vi "FTT Format data.vi"(8 "error in (no error)":errorcluster, 10 "FTT_TV":string, 11 "W/R":bool) -> (0 "error out":errorcluster, 2 "FTT_TV Out":string, 3 "Display":T1)   [LabVIEW 2014]
uses:
  Type'def/Main FTT.ctl
panel:
  # "Plan/Targe(%)"
  # "Taget/Actual"
  # "FTT/FTT(%)"
  # "Repaired/Reject"
  # "/"
  # "/"
  # "/"
  # "/"
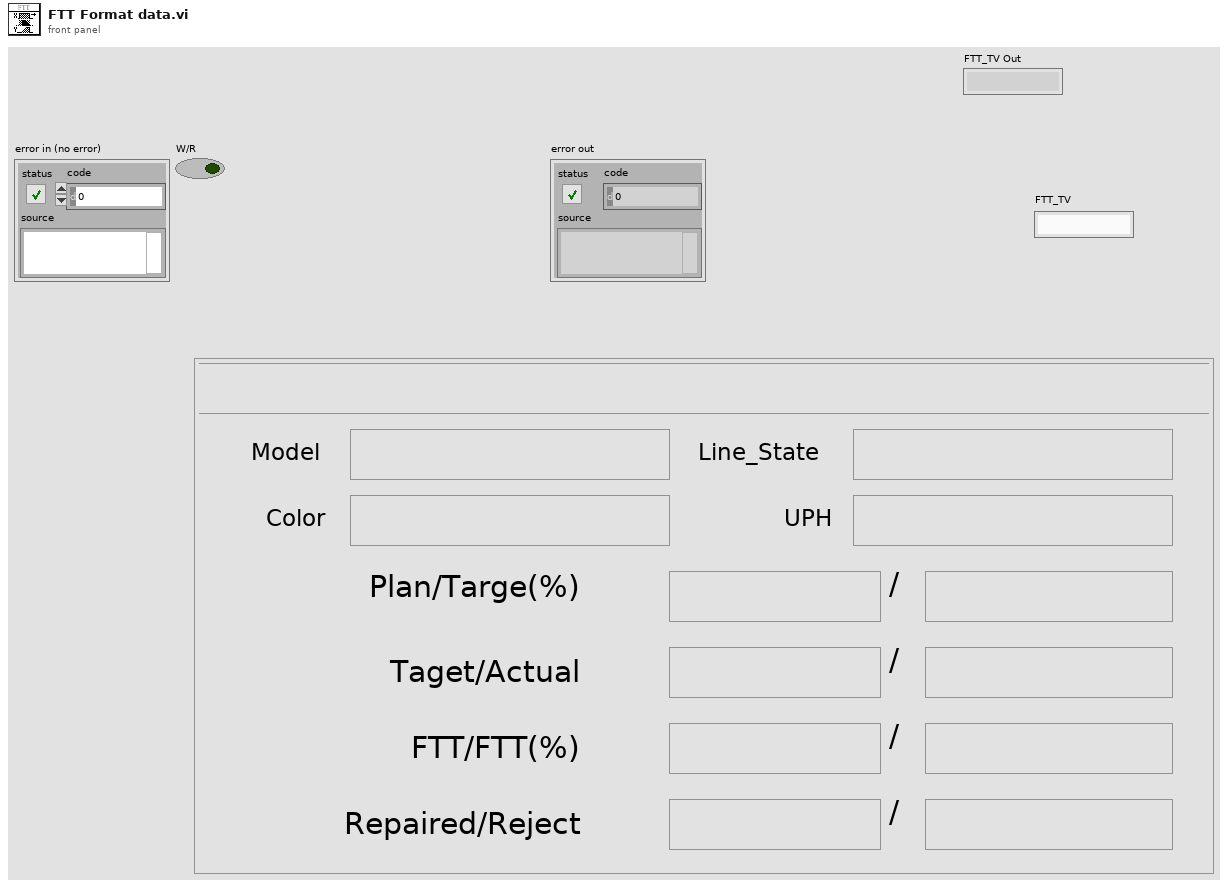
[diagram p1: front panel]
types:
  T1 = typedef "Main FTT.ctl" = cluster{"Line_Name":string, "Model":string, "Line_State":string, "Color":string, "UPH":string, "Plan":string, "Target Rate":string, "Target":string, "Actual":string, "FTT":string, "FTT Rate":string, "Repaired":string, "Reject":string}
  T2 = typedef "FTT Display Type.ctl" = cluster{"Line.No":string, "Model":string, "Color":string, "UPH":dbl, "Plan":dbl, "Target Rate":dbl, "Target ":dbl, "Actual":dbl, "FTT":dbl, "FTT Rate":dbl, "Repaired":dbl, "Reject":dbl, "Ouline":dbl, "Line State":string}
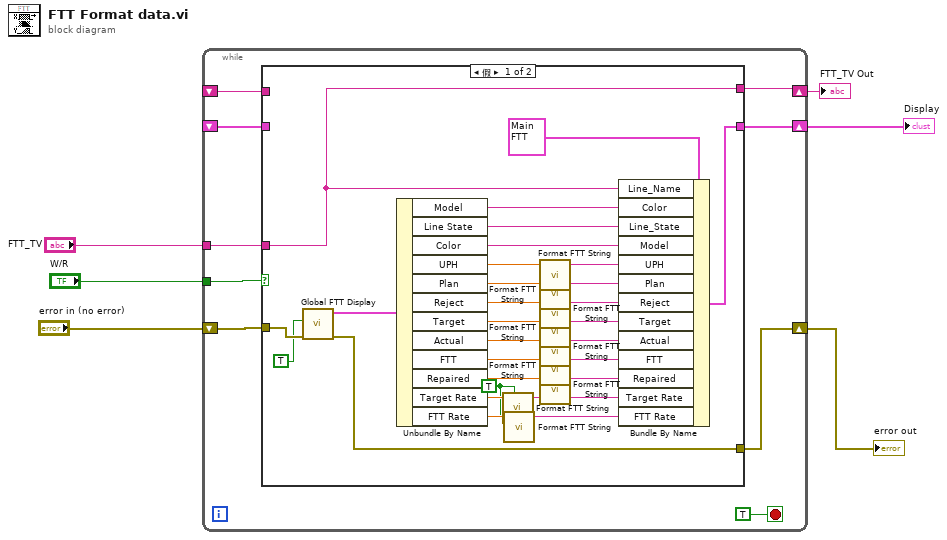
[diagram p0: block diagram]
diagram:
  n1 = while {
    shift-right: [w14] -> w5
    shift-left: "error in (no error)" -> [w15]
    shift-right: [w13] -> w4
    shift-left: _ -> [w12]
    tunnel: "W/R" -> [w11]
    tunnel: "FTT_TV" -> [w9]
    shift-right: [w8] -> w1
    shift-left: _ -> [w7]
    stop <- TRUE stop-if-true
    n2 = case shown="假" w11 {
      tunnel: w15 -> [w42 w47]
      tunnel: [w41 w47] -> w14
      tunnel: [w40 w46] -> w13
      tunnel: w12 -> [_ w46]
      tunnel: w9 -> [w17 _]
      tunnel: [w17 w45] -> w8
      tunnel: w7 -> [_ w45]
      frame False {
        w18 = TRUE
        n3 = call "Global FTT Display.vi"("error in (no error)"=w42, "W/R"=TRUE) -> ("error out"=w41:errorcluster, "Display OUT"=w43:T2)  [unwired: 8 in]
        n4 = Unbundle By Name(w43) -> ("Model"=w39:string, "Line State"=w38:string, "Color"=w37:string, "UPH"=w34:dbl, "Plan"=w32:dbl, "Reject"=w30:dbl, "Target"=w28:dbl, "Actual"=w21:dbl, "FTT"=w22:dbl, "Repaired"=w23:dbl, "Target Rate"=w26:dbl, "FTT Rate"=w35:dbl)
        n5 = call "Format FTT String.vi"("Num in"=w26, "Use Rate?"=w18) -> ("Num out"=w25:string)  [unwired: 5 in]
        n6 = call "Format FTT String.vi"("Num in"=w35, "Use Rate?"=w18) -> ("Num out"=w36:string)  [unwired: 5 in]
        n7 = call "Format FTT String.vi"("Num in"=w34) -> ("Num out"=w33:string)  [unwired: 6 in]
        n8 = call "Format FTT String.vi"("Num in"=w32) -> ("Num out"=w31:string)  [unwired: 6 in]
        n9 = call "Format FTT String.vi"("Num in"=w30) -> ("Num out"=w29:string)  [unwired: 6 in]
        n10 = call "Format FTT String.vi"("Num in"=w28) -> ("Num out"=w27:string)  [unwired: 6 in]
        n11 = call "Format FTT String.vi"("Num in"=w21) -> ("Num out"=w20:string)  [unwired: 6 in]
        n12 = call "Format FTT String.vi"("Num in"=w22) -> ("Num out"=w19:string)  [unwired: 6 in]
        n13 = call "Format FTT String.vi"("Num in"=w23) -> ("Num out"=w24:string)  [unwired: 6 in]
        n14 = Bundle By Name(cluster=T1 {"Line_Name"="TP3 FTT", "Model"="", "Line_State"="", "Color"="", "UPH"="", "Plan"="", "Target Rate"="", "Target"="", "Actual"="", "FTT"="", "FTT Rate"="", "Repaired"="", "Reject"=""} ("Display"), "Line_Name"=w17, "Color"=w39, "Line_State"=w38, "Model"=w37, "UPH"=w33, "Plan"=w31, "Reject"=w29, "Target"=w27, "Actual"=w20, "FTT"=w19, "Repaired"=w24, "Target Rate"=w25, "FTT Rate"=w36) -> (w40:T1)
      }
      frame True {
      }
    }
  }
  "Display" <- w4
  "error out" <- w5
  "FTT_TV Out" <- w1
